vi "calcTimeBase.vi"(11 "time":dbl) -> (2 "base_calculated":u16(ring) items=["ns", "us", "ms"], 3 "time_calculated":u32)   [LabVIEW 2020, in "Camera.lvclass"]
uses:
  Camera.lvclass
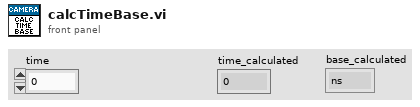
[diagram p1: front panel]
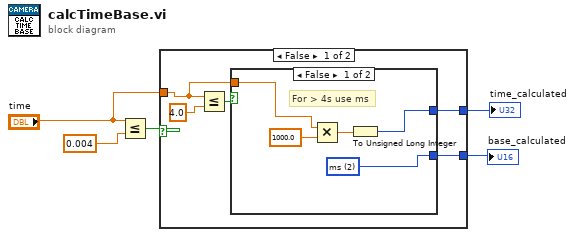
[diagram p0: block diagram]
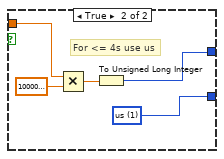
[diagram p2: hidden frame]
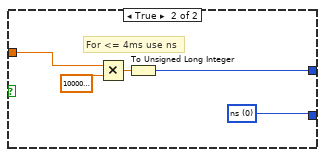
[diagram p3: hidden frame]
diagram:
  n1 = Less Or Equal?(x="time", y=0.004) -> (x <= y?=w4:bool)
  n2 = case shown="False" w4 {
    tunnel: "time" -> [w8 w25]
    tunnel: [w7 w22] -> w2
    tunnel: [w6 w21] -> w1
    frame False {
      n3 = Less Or Equal?(x=w8, y=4.0) -> (x <= y?=w9:bool)
      n4 = case shown="False" w9 {
        tunnel: w8 -> [w13 w20]
        tunnel: [w12 w17] -> w7
        tunnel: [w11 w16] -> w6
        frame False {
          w11 = u16 2 items=["ns", "us", "ms"] ("exposure_time_base")
          # "For > 4s use ms"
          n5 = Multiply(x=w13, y=1000.0) -> (x*y=w15:dbl)
          n6 = To Unsigned Long Integer(number=w15) -> (unsigned 32bit integer=w12:u32)
        }
        frame True {
          w16 = u16 1 items=["ns", "us", "ms"] ("exposure_time_base")
          # "For <= 4s use us"
          n7 = Multiply(x=w20, y=1000000.0) -> (x*y=w18:dbl)
          n8 = To Unsigned Long Integer(number=w18) -> (unsigned 32bit integer=w17:u32)
        }
      }
    }
    frame True {
      w21 = u16 0 items=["ns", "us", "ms"] ("exposure_time_base")
      # "For <= 4ms use ns"
      n9 = Multiply(x=w25, y=1000000000.0) -> (x*y=w23:dbl)
      n10 = To Unsigned Long Integer(number=w23) -> (unsigned 32bit integer=w22:u32)
    }
  }
  "time_calculated" <- w2
  "base_calculated" <- w1
